vi "Sum 3D to 1D.vi"(1 "3D":i32[][][](array[numeric])) -> (0 "1D":i32[](array[numeric]))   [LabVIEW 2009]
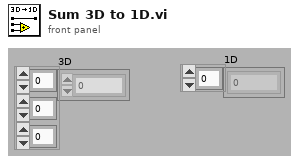
[diagram p1: front panel]
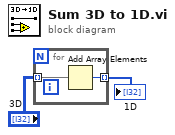
[diagram p0: block diagram]
diagram:
  n1 = for {
    tunnel: "3D" -> [w4] mode=indexing
    tunnel: [w3] -> w2 mode=indexing
    n2 = Add Array Elements(numeric array=w4) -> (sum=w3:i32)
  }
  "1D" <- w2
